vi "Flatten Value.vi"(8 "Error In":errorcluster, 11 "TD Error Cluster In":refnum<class "Error Cluster.lvclass">) -> (0 "Error Out":errorcluster, 1 "Value":string, 3 "TD Error Cluster Out":refnum<class "Error Cluster.lvclass">)   [LabVIEW 2017, in "Tree API.lvlib" / "Error Cluster.lvclass"]
doc: "Dynamic dispatch interface for flattening Tree Data classes to string."
uses:
  Error Cluster.lvclass
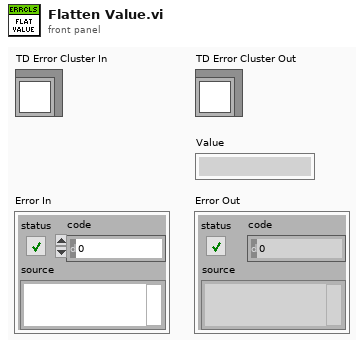
[diagram p1: front panel]
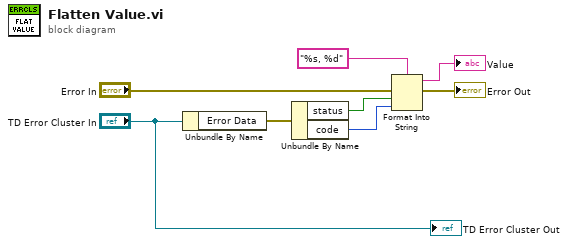
[diagram p0: block diagram]
diagram:
  n1 = Unbundle By Name("TD Error Cluster In") -> ("Error Data"=w7:errorcluster)
  n2 = Unbundle By Name(w7) -> ("status"=w6:bool, "code"=w5:i32)
  n3 = Format Into String(format string="%s, %d", error in="Error In", w6, w5) -> (resulting string=→"Value":string, error out=→"Error Out":errorcluster)  [unwired: 1 in]
  "TD Error Cluster Out" <- "TD Error Cluster In"
